vi "acquis_base_2015-lieto.vi"() -> ()   [LabVIEW 2014]
uses:
  <vilib>/DAQmx/read.llb/DAQmx Read (Analog Wfm 1Chan NSamp).vi
  <vilib>/DAQmx/create/channels.llb/DAQmx Create Channel (AI-Voltage-Basic).vi
  <vilib>/DAQmx/configure/timing.llb/DAQmx Timing (Sample Clock).vi
  <vilib>/DAQmx/miscellaneous.llb/DAQmx Fill In Error Info.vi
  <vilib>/Waveform/WDTFileIO.llb/Export Waveform To Spreadsheet File.vi
panel:
  in  "SALVA I DATI SU FILE":bool=TRUE caption="ON\nOFF"
  out "Waveform Graph":waveform(dbl)(graph)
  in  "Campioni al secondo":dbl=10000.0
  in  "Durata (s)":dbl=0.1
  in  "sample mode":i32(ring)=10178 items=["Finite Samples"=10178, "Continuous Samples"=10123, "Hardware Timed Single Point"=12522]
  in  "physical channels":tag="Dev1/ai0"
  in  "input terminal configuration":i32(ring)=10083 items=["Default"=-1, "RSE"=10083, "NRSE"=10078, "Differential"=10106, "Pseudodifferential"=12529]
  in  "Fondo Scala":dbl(ring)=10.0 items=["10"=10.0, "5"=5.0, "0.5"=0.5, "0.05"=0.05]
  # "NO\nSI"
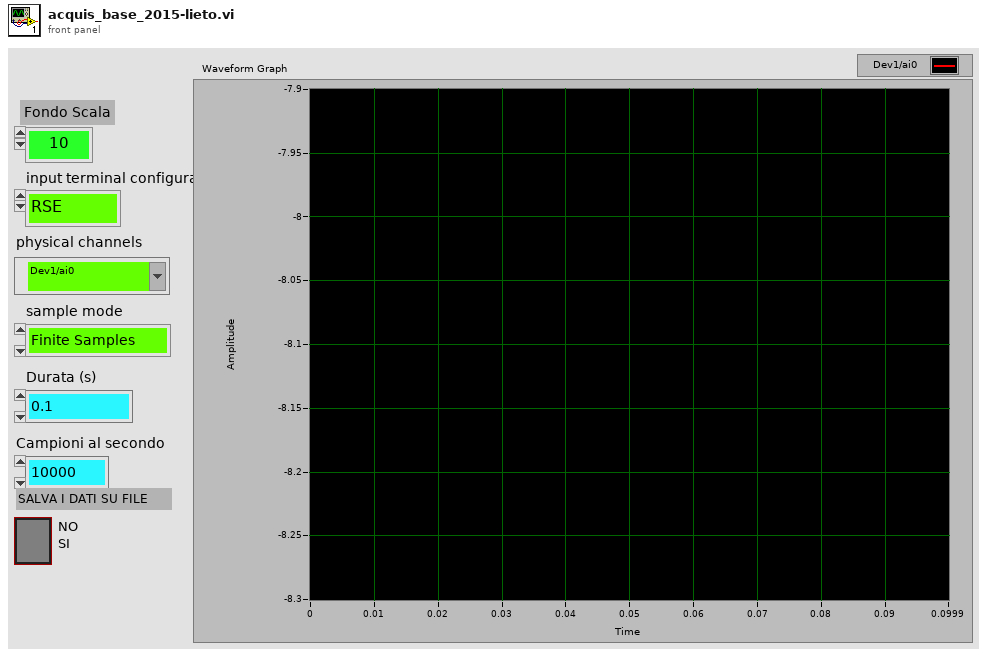
[diagram p1: front panel]
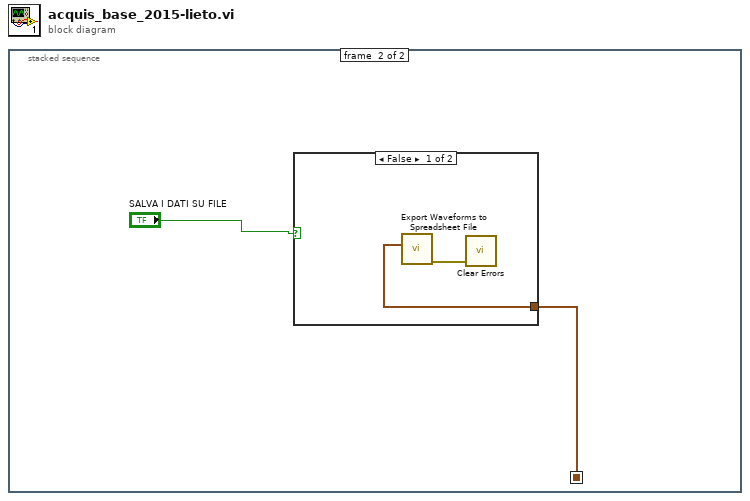
[diagram p0: block diagram]
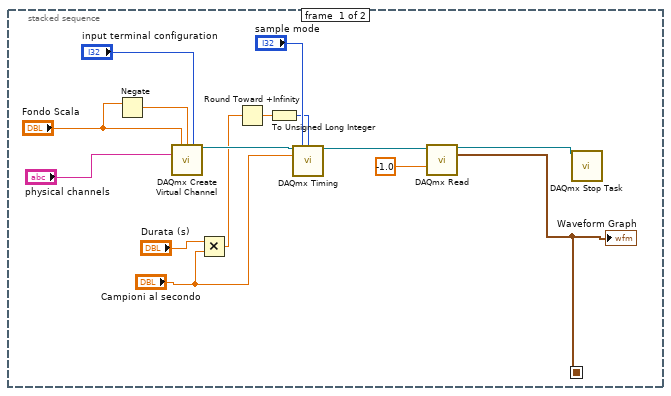
[diagram p2: hidden frame]
diagram:
  n1 = stacked-sequence {
    seq-local: [w1 _] -> [_ w17]
    frame #0 {
      n2 = Negate(x="Fondo Scala") -> (-x=w11:dbl)
      n3 = call-poly <vilib>:"DAQmx Create Virtual Channel.vi"("maximum value"="Fondo Scala", "minimum value"=w11, "input terminal configuration"="input terminal configuration", "physical channels"="physical channels") -> ("task out"=w15:refnum<k21>)  [unwired: 10 in, 1 out]
      n4 = Multiply(x="Durata (s)", y="Campioni al secondo") -> (x*y=w5:dbl)
      n5 = Round Toward +Infinity(x=w5) -> (ceil(x): smallest int >= x=w4:dbl)
      n6 = To Unsigned Long Integer(number=w4) -> (unsigned 32bit integer=w3:u32)
      n7 = call-poly <vilib>:"DAQmx Timing.vi"("task/channels in"=w15, "sample mode"="sample mode", "samples per channel"=w3, "rate"="Campioni al secondo") -> ("task out"=w14:refnum<k21>)  [unwired: 10 in, 1 out]
      n8 = call-poly <vilib>:"DAQmx Read.vi"("task/channels in"=w14, "timeout"=-1.0) -> ("task out"=w13:refnum<k21>, "data"=w1:waveform(dbl))  [unwired: 11 in, 1 out]
      "Waveform Graph" <- w1
      n9 = call <vilib>:"DAQmx Stop Task.vi"("task/channels in"=w13) -> ()  [unwired: 13 in, 2 out]
    }
    frame #1 {
      n10 = case shown="False" "SALVA I DATI SU FILE" {
        tunnel: w17 -> [w19 _]
        frame False {
          n11 = call-poly <vilib>:"Export Waveforms to Spreadsheet File.vi"("waveform"=w19) -> ("error out"=w18:errorcluster)  [unwired: 9 in, 1 out]
          n12 = call <vilib>:"Clear Errors.vi"("error in (no error)"=w18) -> ()  [unwired: 5 in, 2 out]
        }
        frame True {
        }
      }
    }
  }
